vi "Pre Launch Init.vi"(11 "Class Loader in":refnum<class "Class Loader.lvclass">) -> (0 "error out":errorcluster, 3 "Class Loader out":refnum<class "Class Loader.lvclass">)   [LabVIEW 2023, in "Class Loader.lvlib" / "Class Loader.lvclass"]
doc: "(<B>Filename</B>: Actor Framework.lvlib:Actor.lvclass:Pre Launch Init.vi)\n\nDefines behavior that occurs after the Launch Nested Actor method is invoked but before the actor's Actor Core method begins running.\n\nBy default, this method does nothing. A descendant class may override it to define behavior."
uses:
  Class Loader.lvclass
  Class Loader.lvclass/Class Loader.ctl
  <vilib>/ActorFramework/Message Enqueuer/Message Enqueuer.lvclass
  Load Inputs.ctl
  <vilib>/LS Instruments AG/Async Methods Actor/Async Methods Actor/Async Methods Actor/Async Methods Actor.lvclass
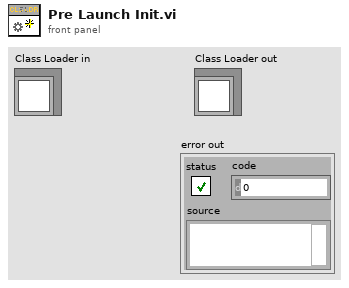
[diagram p1: front panel]
types:
  T1 = typedef "Class Loader.lvlib/Class Loader.lvclass/Load Inputs.ctl" = cluster{"Caller Enqueuer":refnum<class "Message Enqueuer.lvclass">, "Reference Class Path":path, "Class Relative Paths Path":path}
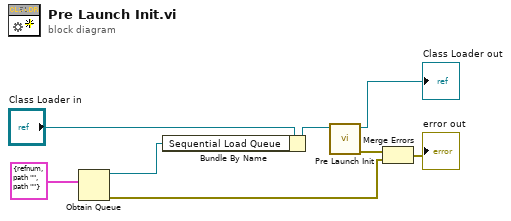
[diagram p0: block diagram]
diagram:
  n1 = Obtain Queue(element data type=T1 {"Caller Enqueuer"=refnum, "Reference Class Path"=path "", "Class Relative Paths Path"=path ""} ("Load Inputs")) -> (queue out=w3:refnum<queue>, error out=w1:errorcluster)  [unwired: 4 in, 1 out]
  n2 = Bundle By Name(cluster="Class Loader in", "Sequential Load Queue"=w3) -> (w4:refnum<class "Class Loader.lvclass">)
  n3 = call-parent "Pre Launch Init.vi"("Async Methods Actor in"=w4) -> ("error out"=w8:errorcluster, "Async Methods Actor out"=→"Class Loader out":refnum<class "Class Loader.lvclass">)  [unwired: 9 in]
  n4 = Merge Errors(w8, w1) -> (→"error out":errorcluster)
